vi "Lift Control Logic.vi"(0 "Operator Gamepad":T1, 5 "Limit Switches":T8, 7 "Lift Potentiometer":T9={"DevStatus"={"status"=FALSE, "code"=0, "source"=""}, "Controller"=enum."Controller 1", "Analog Channel"=enum."Invalid", "Invert Output"=FALSE}, 9 "Gripper Encoder":T12={"DevStatus"={"status"=FALSE, "code"=0, "source"=""}, "EncoderIndex"=enum."Invalid", "CounterIndex"=enum."Invalid", "DistancePerCount"=1.0, "Decoding Type"=enum."4x"}, 12 "Gripper Gains":cluster{"P":dbl, "I":dbl, "D":dbl}, 13 "Manual?":bool, 14 "PID/Profiler":bool) -> (6 "State Out":T3(ring), 8 "Done?":bool, 10 "Lift Motor":dbl, 15 "Gripper":dbl)   [LabVIEW 2014]
uses:
  <vilib>/Rock Robotics/WPI/Encoder/WPI_EncoderDevRef.ctl
  <vilib>/Rock Robotics/SystemInterfaces/Encoder/FPGA_EncoderIdx.ctl
  <vilib>/Rock Robotics/SystemInterfaces/Counter/FPGA_CounterCtrSystemIndex.ctl
  <vilib>/Rock Robotics/WPI/Encoder/WPI_EncoderType.ctl
  <vilib>/Rock Robotics/WPI/Potentiometer/WPI_PotentiometerDevRef.ctl
  <vilib>/Rock Robotics/SystemInterfaces/Typedef/FPGA_TypedefAnalogModule.ctl
  <vilib>/Rock Robotics/SystemInterfaces/AI/FPGA_AIChannel.ctl
  <vilib>/Rock Robotics/WPI/Switch/WPI_SwitchDevRef.ctl
  <vilib>/Rock Robotics/SystemInterfaces/DIO/FPGA_DIOChannel.ctl
  <vilib>/Rock Robotics/SystemInterfaces/Typedef/FPGA_TypedefDigitalModule.ctl
  <vilib>/Rock Robotics/WPI/Joystick/WPI_JoystickDevRef.ctl
  <vilib>/Rock Robotics/WPI/Joystick/WPI_JoystickDeviceEnum.ctl
panel:
  in  "Lift Gains":cluster{"P":dbl, "I":dbl, "D":dbl}={"P"=0.24, "I"=5.6e-07, "D"=0.0}
  in  "State":T3(ring)=enum."Override"
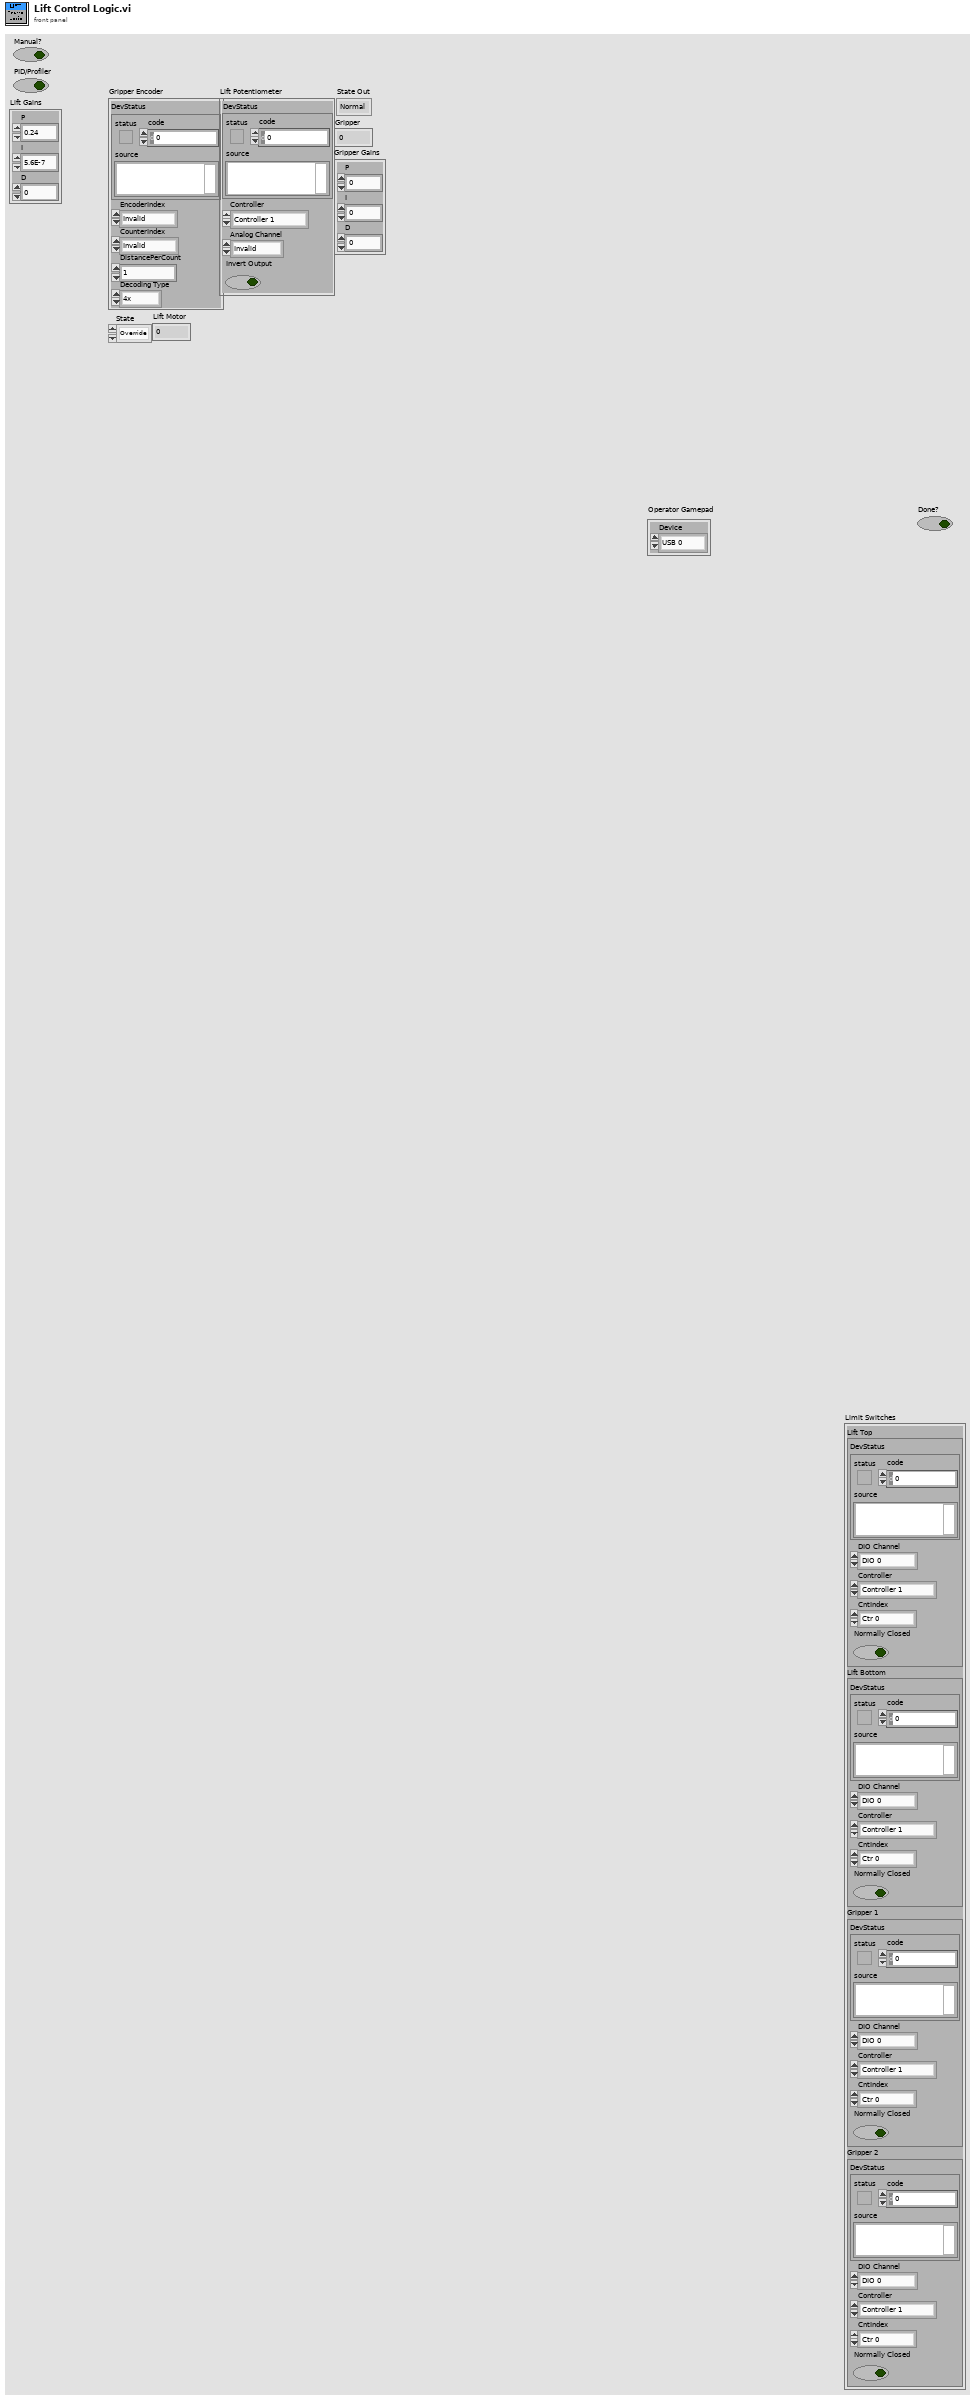
[diagram p1: front panel]
types:
  T1 = typedef "WPI_JoystickDevRef.ctl" = cluster{"Device":T2}
  T2 = typedef "WPI_JoystickDeviceEnum.ctl" = enum16{"USB 0", "USB 1", "USB 2", "USB 3", "USB 4", "USB 5"}
  T3 = enum16{"Normal", "Down/Out", "Down/In", "Up", "Override"}
  T4 = typedef "WPI_SwitchDevRef.ctl" = cluster{"DevStatus":errorcluster, "DIO Channel":T5, "Controller":T6, "CntIndex":T7, "Normally Closed":bool}
  T5 = typedef "FPGA_DIOChannel.ctl" = enum8{"DIO 0", "DIO 1", "DIO 2", "DIO 3", "DIO 4", "DIO 5", "DIO 6", "DIO 7", "DIO 8", "DIO 9", "DIO MXP 0", "DIO MXP 1", "DIO MXP 2", "DIO MXP 3", "DIO MXP 4", "DIO MXP 5", "DIO MXP 6", "DIO MXP 7", "DIO MXP 8", "DIO MXP 9", "DIO MXP 10", "DIO MXP 11", "DIO MXP 12", "DIO MXP 13", "DIO MXP 14", "DIO MXP 15", "Invalid"}
  T6 = typedef "FPGA_TypedefDigitalModule.ctl" = enum16{"Controller 1"}
  T7 = typedef "FPGA_CounterCtrSystemIndex.ctl" = enum8{"Ctr 0", "Ctr 1", "Ctr 2", "Ctr 3", "Ctr 4", "Ctr 5", "Ctr 6", "Ctr 7", "Invalid"}
  T8 = cluster{"Lift Top":T4, "Lift Bottom":T4, "Gripper 1":T4, "Gripper 2":T4}
  T9 = typedef "WPI_PotentiometerDevRef.ctl" = cluster{"DevStatus":errorcluster, "Controller":T10, "Analog Channel":T11, "Invert Output":bool}
  T10 = typedef "FPGA_TypedefAnalogModule.ctl" = enum16{"Controller 1"}
  T11 = typedef "FPGA_AIChannel.ctl" = enum8{"AI 0", "AI 1", "AI 2", "AI 3", "AI MXP 0", "AI MXP 1", "AI MXP 2", "AI MXP 3", "Invalid"}
  T12 = typedef "WPI_EncoderDevRef.ctl" = cluster{"DevStatus":errorcluster, "EncoderIndex":T13, "CounterIndex":T7, "DistancePerCount":dbl, "Decoding Type":T14}
  T13 = typedef "FPGA_EncoderIdx.ctl" = enum8{"Enc 0", "Enc 1", "Enc 2", "Enc 3", "Enc 4", "Enc 5", "Enc 6", "Enc 7", "Invalid"}
  T14 = typedef "WPI_EncoderType.ctl" = enum16{"1x", "2x", "4x"}
  T15 = cluster{"State Out":enum16{"Normal", "Down/Out", "Down/In", "Up", "Override"}, "To Shift":cluster{"Cluster in":cluster{"Scaled Value Out":dbl, "Distance":dbl}, "To Shift":cluster{"Error":dbl, "millisecond timer value":u32, "To Shift Register":dbl}, "To Shift":dbl}}
  T16 = cluster{"Cluster in":cluster{"Scaled Value Out":dbl, "Distance":dbl}, "To Shift":cluster{"Error":dbl, "millisecond timer value":u32, "To Shift Register":dbl}, "To Shift":dbl}
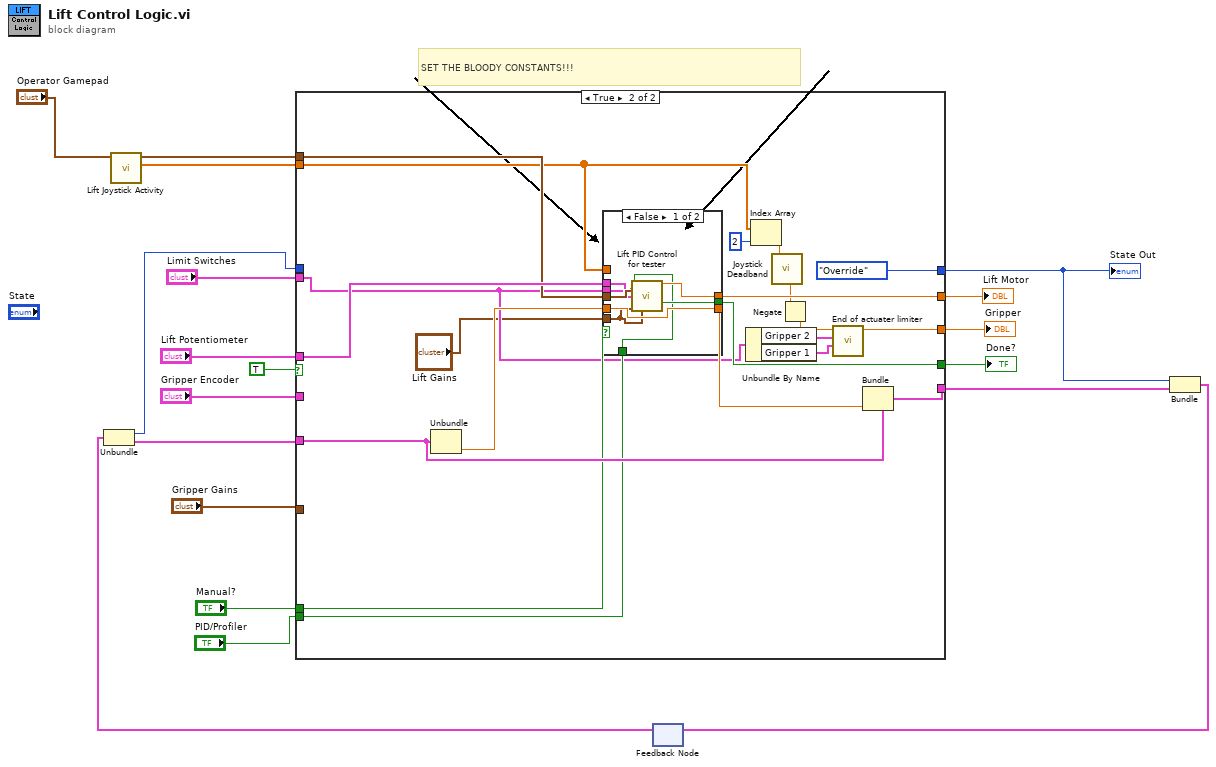
[diagram p0: block diagram]
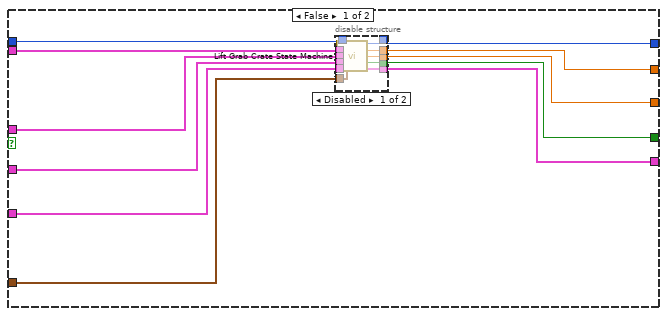
[diagram p2: hidden frame]
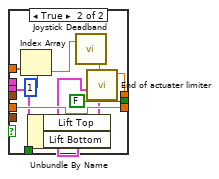
[diagram p4: hidden frame]
diagram:
  # "SET THE BLOODY CONSTANTS!!!"
  n1 = call "Lift Joystick Activity.vi"("Operator Gamepad"="Operator Gamepad") -> ("Axes"=w4:dbl[], "Gamepad Out"=w5:T1)  [unwired: 8 in, 1 out]
  n2 = feedback #1() -> (w7:T15)  [unwired: 1 in]
  n3 = Unbundle(w7) -> ("State Out"=w13:T3, "To Shift"=w16:T16)
  n4 = case shown="True" TRUE ("Boolean") {
    tunnel: "Lift Potentiometer" -> [w27 w59]
    tunnel: [w30 T3."Override"] -> w17
    tunnel: "Gripper Gains" -> [w20 _]
    tunnel: w13 -> [w28 _]
    tunnel: w16 -> [w24 w57]
    tunnel: "Limit Switches" -> [w29 w47]
    tunnel: "Gripper Encoder" -> [w26 _]
    tunnel: [w25 w58] -> w11
    tunnel: [w23 w60] -> w10
    tunnel: [w22 w48] -> w9
    tunnel: [w21 w61] -> w8
    tunnel: w5 -> [_ w54]
    tunnel: w4 -> [_ w52]
    tunnel: "Manual?" -> [_ w51]
    tunnel: "PID/Profiler" -> [_ w50]
    frame False {
      n5 = disable-structure shown="Disabled" {
        disable-tunnel: [w41 _] -> w30
        disable-tunnel: w29 -> [w40 _]
        disable-tunnel: w28 -> [w39 _]
        disable-tunnel: w27 -> [w38 _]
        disable-tunnel: w26 -> [w37 _]
        disable-tunnel: [w36 _] -> w25
        disable-tunnel: w24 -> [w35 _]
        disable-tunnel: [w34 _] -> w23
        disable-tunnel: [w33 _] -> w22
        disable-tunnel: [w32 _] -> w21
        disable-tunnel: w20 -> [w31 _]
        frame Disabled {
          n6 = call "Lift Grab Crate State Machine.vi"("State In"=w39, "Limit Switches"=w40, "Lift Potentiometer"=w38, "Gripper Encoder"=w37, "From Shift"=w35, "Gripper Gains"=w31) -> ("State Out"=w41:T3, "Lift Output"=w32:dbl, "Gripper Output"=w33:dbl, "Done?"=w34:bool, "To Shift"=w36:T16)  [unwired: 5 in]
        }
        frame Enabled {
        }
      }
    }
    frame True {
      n7 = Unbundle(w57) -> ("To Shift"=w55:dbl)  [unwired: 2 out]
      n8 = case shown="False" w51 {
        tunnel: [w69 w76] -> w61
        tunnel: [w70 FALSE ("Tolerable?")] -> w60
        tunnel: w59 -> [w66 _]
        tunnel: w47 -> [w65 w75]
        tunnel: [w68 w77] -> w56
        tunnel: w55 -> [w68 w77]
        tunnel: w54 -> [w67 _]
        tunnel: w52 -> [_ w80]
        tunnel: w50 -> [w64 _]
        tunnel: "Lift Gains" -> [w63 _]
        frame False {
          n9 = call "Lift PID Control for tester.vi"("Use Motion Profiler"=w64, "Limit Switches"=w65, "Operator Gamepad"=w67, "Lift Potentionmeter"=w66, "Gains UP"=w63, "Gains DOWN"=w63) -> ("Motor output"=w69:dbl, "Tolerable?"=w70:bool)  [unwired: 8 in]
        }
        frame True {
          n10 = Index Array(array=w80, index=1) -> (element=w71:dbl)
          n11 = Unbundle By Name(w75) -> ("Lift Top"=w72:T4, "Lift Bottom"=w73:T4)
          n12 = call "Joystick Deadband.vi"("Joystick Value"=w71) -> ("Joystick Output"=w74:dbl)  [unwired: 1 in]
          n13 = call "End of actuater limiter.vi"("Lower limit switch"=w73, "Upper limit switch"=w72, "Motor input"=w74) -> ("Motor output"=w76:dbl)  [unwired: 8 in]
        }
      }
      n14 = Unbundle By Name(w47) -> ("Gripper 2"=w45:T4, "Gripper 1"=w46:T4)
      n15 = Index Array(array=w52, index=2) -> (element=w49:dbl)
      n16 = call "Joystick Deadband.vi"("Joystick Value"=w49) -> ("Joystick Output"=w44:dbl)  [unwired: 1 in]
      n17 = Negate(x=w44) -> (-x=w43:dbl)
      n18 = call "End of actuater limiter.vi"("Lower limit switch"=w46, "Upper limit switch"=w45, "Motor input"=w43) -> ("Motor output"=w48:dbl)  [unwired: 8 in]
      n19 = Bundle(cluster=w57, "To Shift"=w56) -> (w58:T16)  [unwired: 2 in]
    }
  }
  "Gripper" <- w9
  "State Out" <- w17
  "Lift Motor" <- w8
  "Done?" <- w10
  n20 = Bundle("State Out"=w17, "To Shift"=w11) -> (w15:T15)  [unwired: 1 in]
  n21 = feedback-in #1(w15) -> ()
